vi "getBranch.vi"(11 "gitStatusResponse":string) -> (3 "branch":string)   [LabVIEW 2023, in "gitTools.lvlib"]
uses:
  gitTools.lvlib
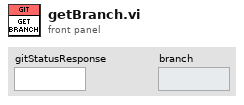
[diagram p1: front panel]
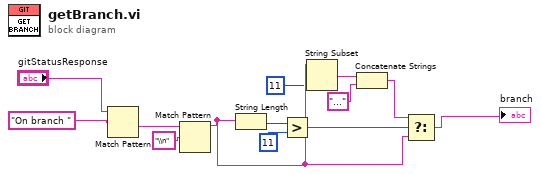
[diagram p0: block diagram]
diagram:
  n1 = Match Pattern(string="gitStatusResponse", regular expression="On branch ") -> (after substring=w4:string)  [unwired: 1 in, 3 out]
  n2 = Match Pattern(string=w4, regular expression="\\n") -> (before substring=w12:string)  [unwired: 1 in, 3 out]
  n3 = String Length(string=w12) -> (length=w6:i32)
  n4 = Greater?(x=w6, y=11) -> (0:w8:bool)
  n5 = String Subset(string=w12, length (rest)=11 ("length (rest)")) -> (substring=w9:string)  [unwired: 1 in]
  n6 = Concatenate Strings(w9, "..." ("string")) -> (w11:string)
  n7 = Select(t=w11, s=w8, f=w12) -> (s? t:f=→"branch":string)
